vi "get gear settings.vi"(8 "error in (no error)":errorcluster, 10 "gear_settings":T1, 11 "id":i32) -> (0 "error out":errorcluster, 2 "gear_settings out":T1, 3 "function return":i32)   [LabVIEW 2012, in "libximc.lvlib"]
doc: "result_t XIMC_API get_gear_settings (device_t id, gear_settings_t* gear_settings);"
uses:
  libximc.lvlib
  libximc.dll
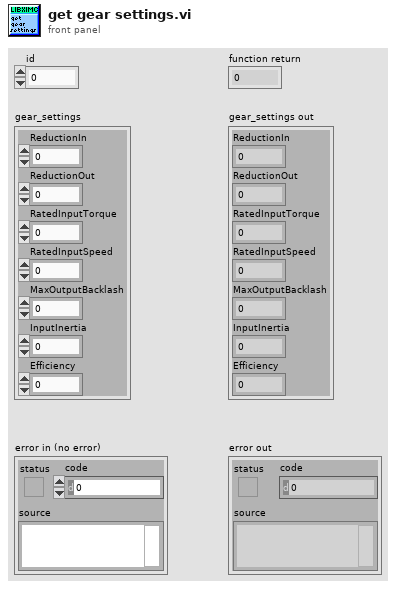
[diagram p1: front panel]
types:
  T1 = cluster{"ReductionIn":sgl, "ReductionOut":sgl, "RatedInputTorque":sgl, "RatedInputSpeed":sgl, "MaxOutputBacklash":sgl, "InputInertia":sgl, "Efficiency":sgl}
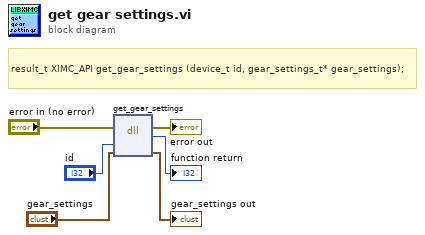
[diagram p0: block diagram]
diagram:
  # "result_t XIMC_API get_gear_settings (device_t id, gear_settings_t* gear_settings);"
  n1 = dll-call lib="E:/labview-2.12.1-Labview_12.0/ximcLVx32/libximc.*" fn="get_gear_settings"(error in="error in (no error)", "id"="id", "gear_settings"="gear_settings") -> (error out=→"error out":errorcluster, →"function return":i32, "gear_settings"=→"gear_settings out":T1)  [unwired: 3 in, 1 out]
